vi "CLSUIP_GetControlPosition.vi"(8 "error in (no error)":errorcluster, 11 "VI Refnum":refnum<vi>) -> (0 "error out":errorcluster, 2 "Position":T1, 3 "VI Refnum out":refnum<vi>)   [LabVIEW 2021, in "MemberVICreation.lvlib"]
uses:
  <resource>/Framework/Providers/LVClassLibrary/NewAccessors/MemberVICreation.lvlib
  <vilib>/Utility/miscctls.llb/LVPositionTypeDef.ctl
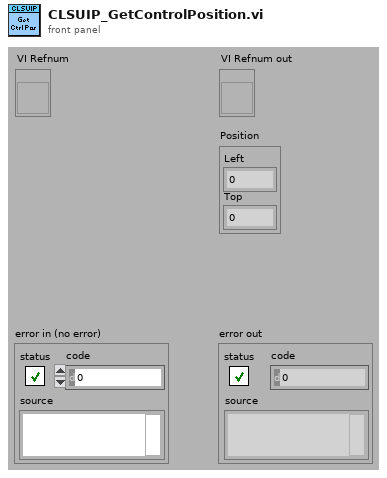
[diagram p1: front panel]
types:
  T1 = typedef "LVPositionTypeDef.ctl" = cluster{"Left":i32, "Top":i32}
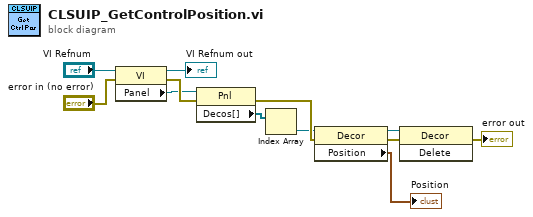
[diagram p0: block diagram]
diagram:
  n1 = property class="VI"(reference="VI Refnum", error in="error in (no error)") -> (reference out=→"VI Refnum out":refnum<vi>, error out=w11:errorcluster, "Panel"=w10:refnum<vi>)
  n2 = property class="Pnl"(reference=w10, error in=w11) -> (error out=w9:errorcluster, "Decos[]"=w7:refnum<vi>[])  [unwired: 1 out]
  n3 = Index Array(array=w7) -> (element=w6:refnum<vi>)  [unwired: 1 in]
  n4 = property class="Decor"(reference=w6, error in=w9) -> (reference out=w4:refnum<vi>, error out=w3:errorcluster, "Position"=→"Position":T1)
  n5 = invoke class="Decor" method="Delete"(reference=w4, error in=w3) -> (error out=→"error out":errorcluster)  [unwired: 1 in, 2 out]
